vi "Handle Error.vi"(8 "error in (no error)":errorcluster, 11 "Caller in":refnum<class "Caller.lvclass">) -> (0 "error out":errorcluster, 2 "stop actor?":bool=TRUE, 3 "Caller out":refnum<class "Caller.lvclass">)   [LabVIEW 2020, in "Caller.lvlib" / "Caller.lvclass"]
doc: "(<B>Filename</B>: Actor Framework.lvlib:Actor.lvclass:Handle Error.vi)\n\nDefines how the actor handles an error that occurred while processing a message. By default, this method does nothing except stop the actor."
uses:
  Caller.lvclass
  <vilib>/ActorFramework/Actor/Actor.lvclass
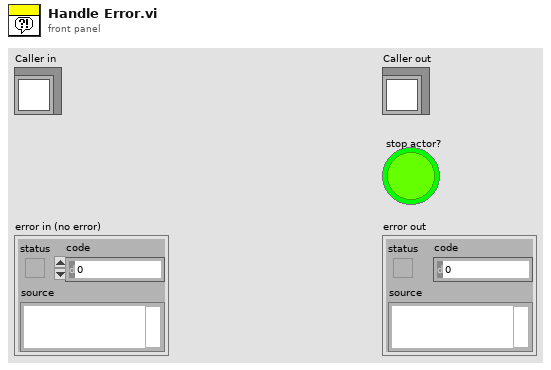
[diagram p1: front panel]
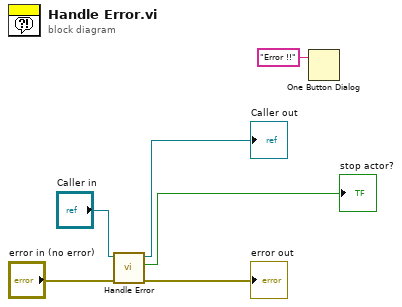
[diagram p0: block diagram]
diagram:
  n1 = call-parent "Handle Error.vi"("error in (no error)"="error in (no error)", "Actor in"="Caller in") -> ("error out"=→"error out":errorcluster, "stop actor?"=→"stop actor?":bool, "Actor out"=→"Caller out":refnum<class "Caller.lvclass">)  [unwired: 7 in]
  n2 = One Button Dialog(message="Error !!") -> ()  [unwired: 1 in, 1 out]
